vi "Main.vi"() -> ()   [LabVIEW 2020]
doc: "This template is for the Queued Message Handler design pattern.\n\nThe Event Handling Loop generates messages based on user interface actions.\n\nThe Message Handling Loop processes messages generated by the Event Handling Loop, or by other messages. The messages are string values, so new messages can be added easily to the Message Cases case structure in the Message Handling Loop. Each message cluster can also provide an optional value for Message Data, which is a variant that can be converted to whatever message-specific data is required."
uses:
  TrioMotion Controller/Connection Type.ctl
  support/Message Queue/Message Cluster.ctl
  controls/MHL Data.ctl
  controls/MHL UI Data.ctl
  controls/MHL Status.ctl
  controls/MHL References.ctl
  controls/MHL Configuration.ctl
  <extravilib>/ChannelInstances/Messenger-t'Message Queue.lvlib-Message Cluster.ctl'/Write With Abort.vi
  <extravilib>/ChannelInstances/Messenger-t'Message Queue.lvlib-Message Cluster.ctl'/Instantiate.vi
  <extravilib>/ChannelInstances/Messenger-t'Message Queue.lvlib-Message Cluster.ctl'/Endpoint.vi
  <extravilib>/ChannelInstances/Event Messenger-bool/Instantiate.vi
  <extravilib>/ChannelInstances/Event Messenger-bool/))Channel.vi
  <vilib>/Utility/error.llb/Error Cluster From Error Code.vi
  <vilib>/ErrorRing/Error Ring.xnode
  <extravilib>/ChannelInstances/Event Messenger-bool.lvlib
  support/Message Queue/Message Queue.lvlib
  <extravilib>/ChannelInstances/Messenger-t'Message Queue.lvlib-Message Cluster.ctl'.lvlib
  TrioMotion Controller/TrioMotion Controller.lvlib
panel:
  in  "Home Axes":bool
  in  "Enable Axes":bool
  in  "Set Parameters":bool
  in  "Connection Type":T1
  in  "Connect to Controller":bool
  out "Status":string
  in  "Exit":bool
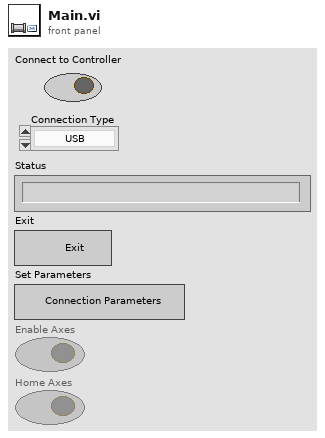
[diagram p1: front panel]
types:
  T1 = typedef "TrioMotion Controller.lvlib/Connection Type.ctl" = enum16{"USB", "Serial", "Ethernet", "PCI", "Path", "No connection"}
  T2 = typedef "MHL Data.ctl" = cluster{"MHL UI Data":T3, "MHL References":T5, "MHL Configuration":T6}
  T3 = typedef "MHL UI Data.ctl" = cluster{"Status":string, "Connection Type":T1, "Connected to Controller":bool, "Axes Enabled":bool, "Jogging Enabled":bool, "X Axis MPOS":dbl, "A Axis MPOS":dbl, "X Axis SPEED":dbl, "A Axis SPEED":dbl, "Plot Laser Data":bool, "MHL Status":T4}
  T4 = typedef "MHL Status.ctl" = enum16{"Disconnected", "Connecting", "Connected", "Axes Enabled", "Machine Running", "Shutdown"}
  T5 = typedef "MHL References.ctl" = cluster{"Connect to Controller Ref":refnum<vi>, "Connection Type Ref":refnum<vi>, "Set Parameters Ref":refnum<vi>, "Enable Axes Ref":refnum<vi>, "Home Axes Ref":refnum<vi>}
  T6 = typedef "MHL Configuration.ctl" = cluster{"Fuel Control Valve Maximum":dbl, "Fuel Control Valve Minimum":dbl}
  T7 = typedef "Message Queue.lvlib/Message Cluster.ctl" = cluster{"Message":string, "Message Data":variant}
  T8 = typedef "Notifiers.ctl" = cluster{"Handshake":refnum<notifier>, "Connection Established":refnum<notifier>, "Controller Exit":refnum<notifier>}
  T9 = typedef "Messenger-t'Message Queue.lvlib-Message Cluster.ctl'.lvlib/))Channel.ctl" = refnum<queue>
  T10 = typedef "Event Messenger-bool.lvlib/))Channel.ctl" = refnum<queue>
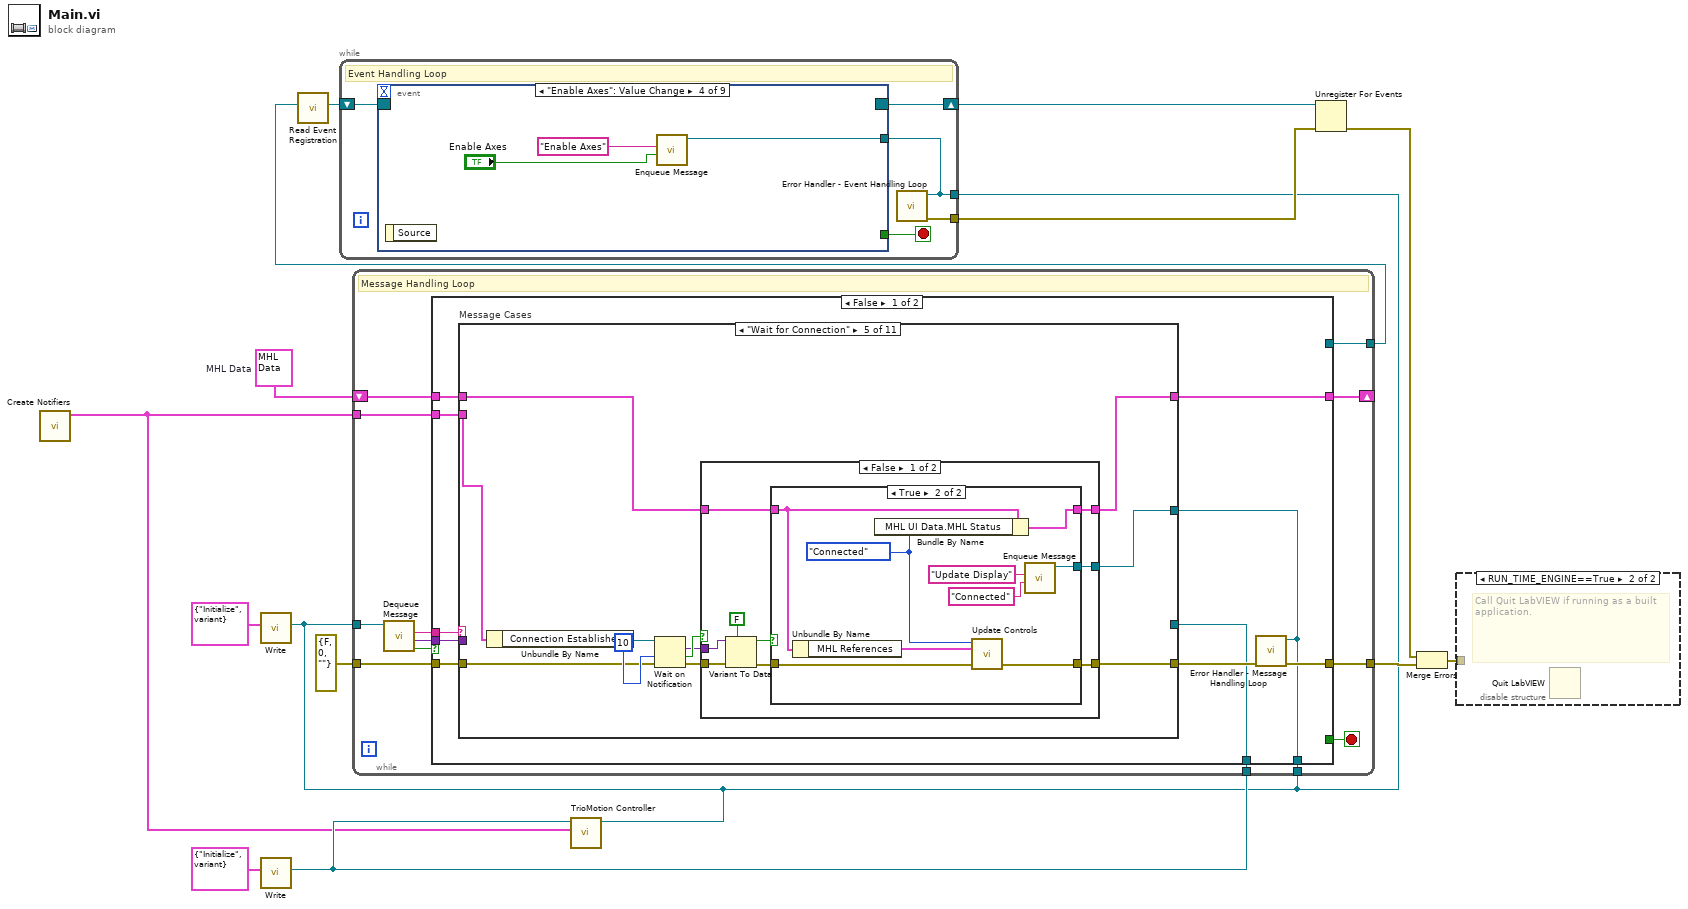
[diagram p0: block diagram]
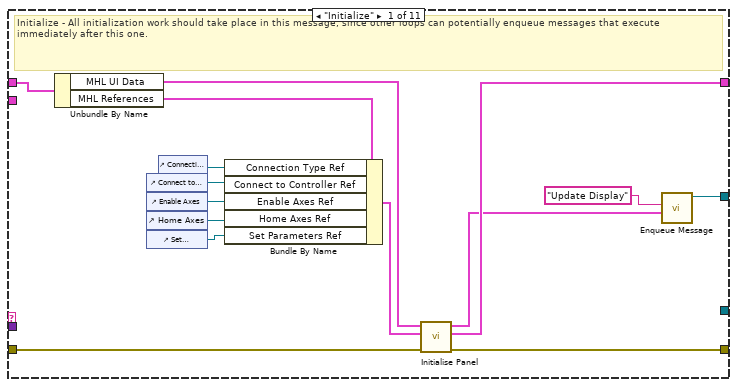
[diagram p2: hidden frame]
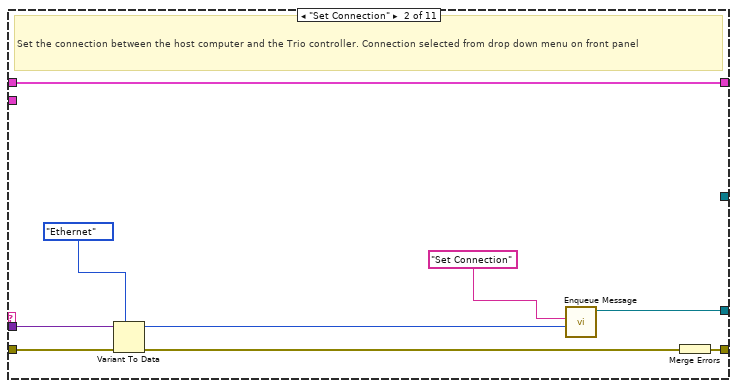
[diagram p3: hidden frame]
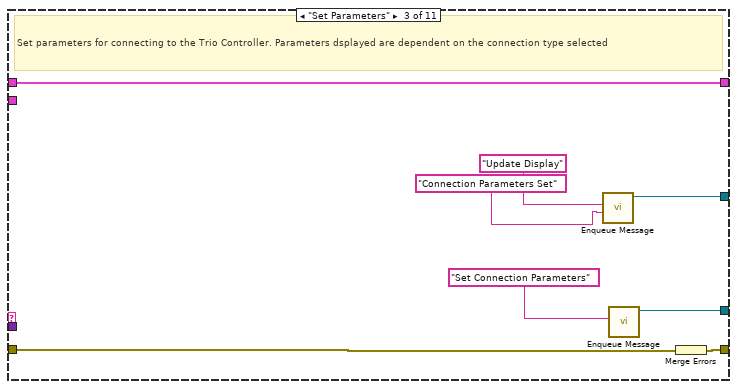
[diagram p4: hidden frame]
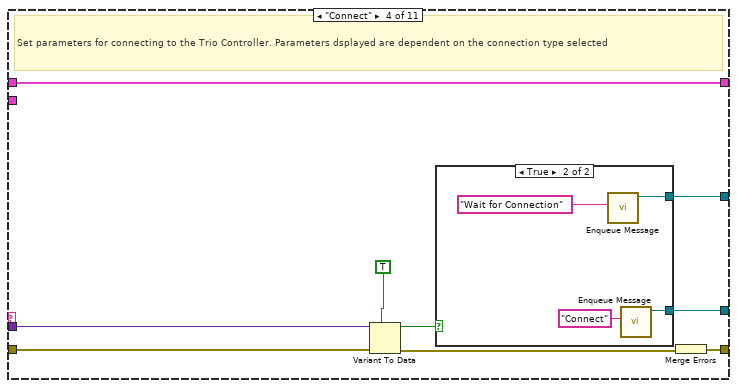
[diagram p5: hidden frame]
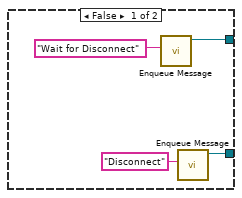
[diagram p6: hidden frame]
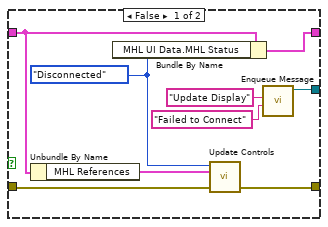
[diagram p7: hidden frame]
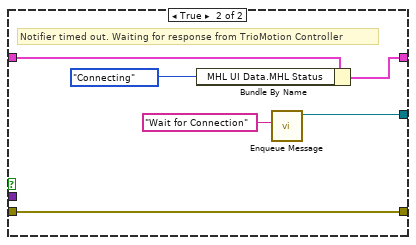
[diagram p8: hidden frame]
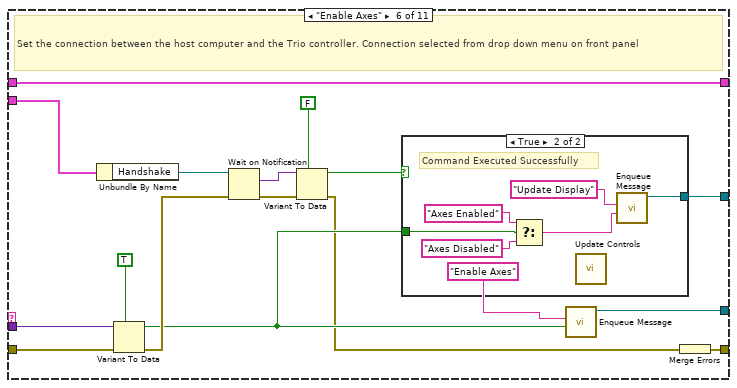
[diagram p9: hidden frame]
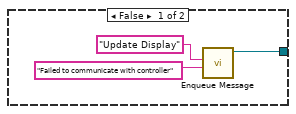
[diagram p10: hidden frame]
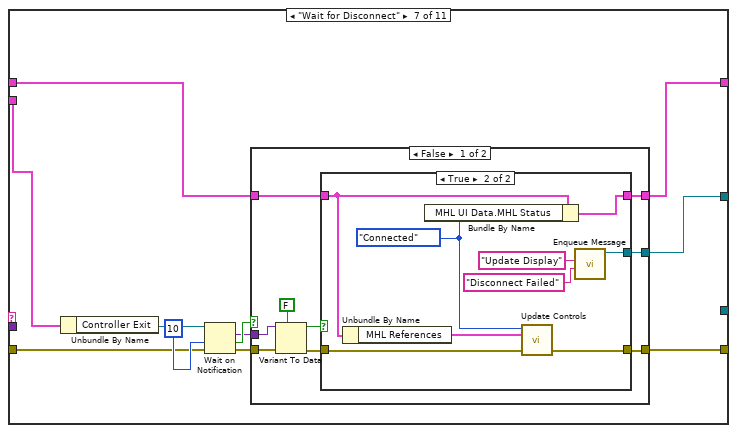
[diagram p11: hidden frame]
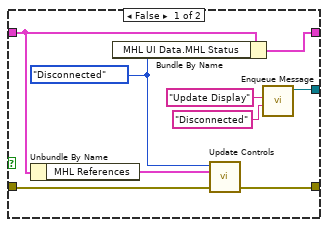
[diagram p12: hidden frame]
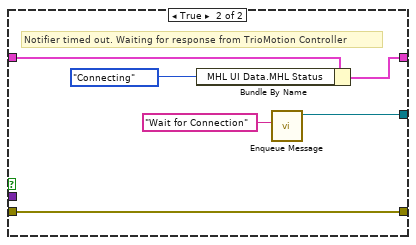
[diagram p13: hidden frame]
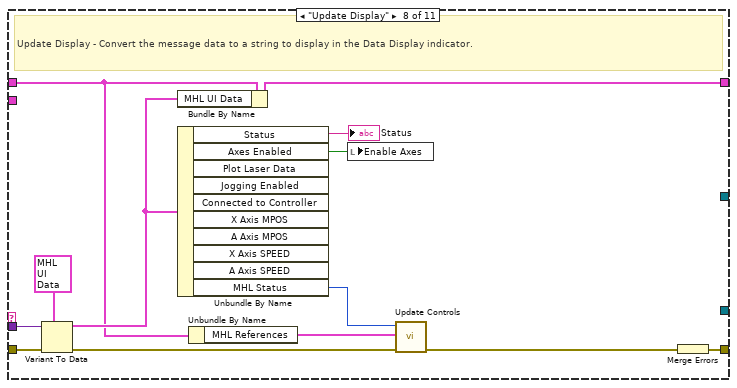
[diagram p14: hidden frame]
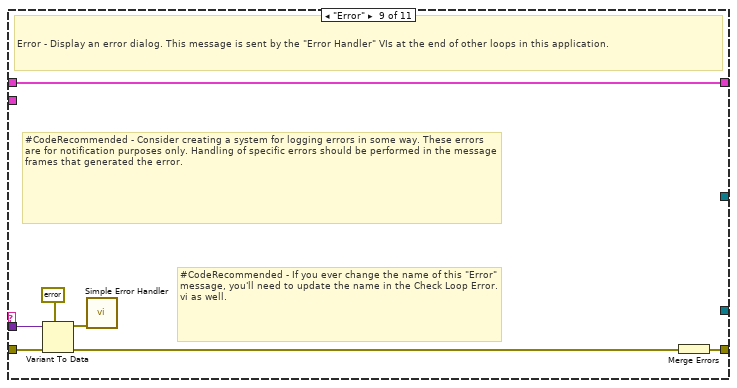
[diagram p15: hidden frame]
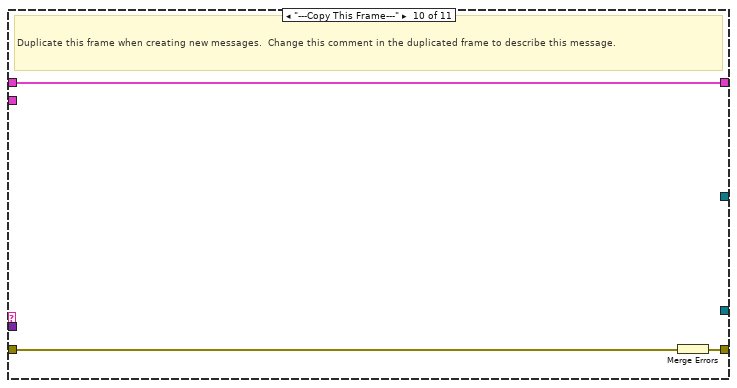
[diagram p16: hidden frame]
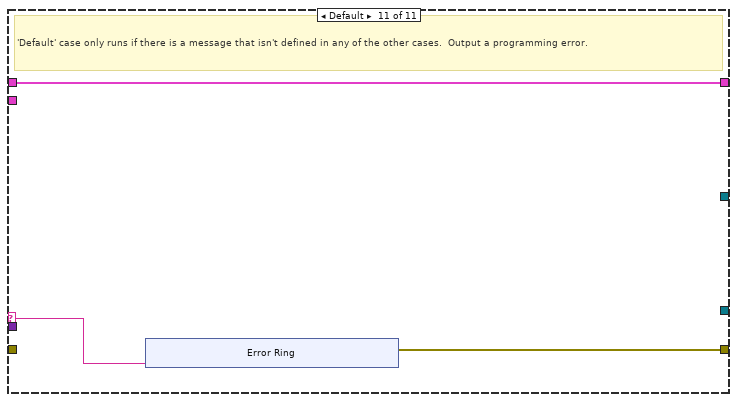
[diagram p17: hidden frame]
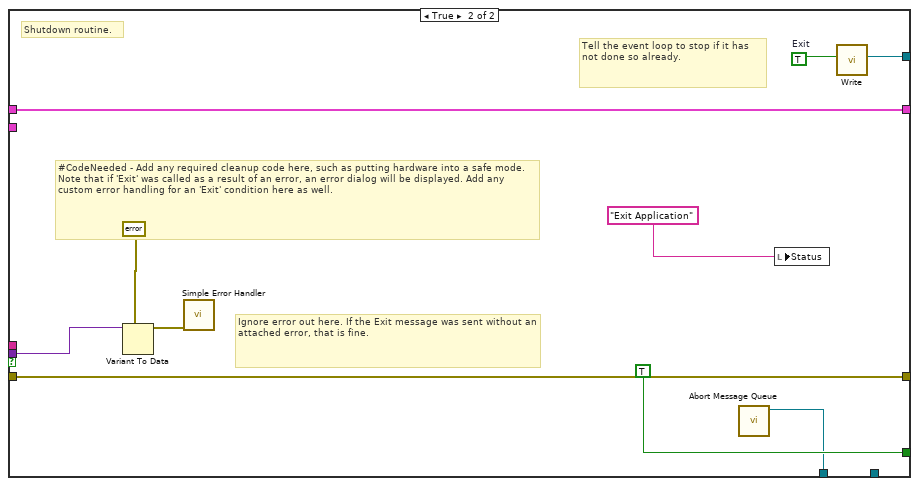
[diagram p18: hidden frame]
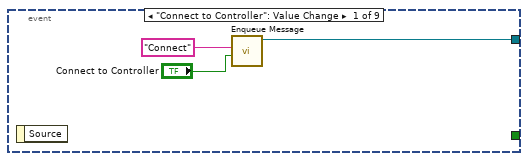
[diagram p20: hidden frame]
diagram:
  w3 = T2 {"MHL UI Data"={"Status"="", "Connection Type"=enum."Ethernet", "Connected to Controller"=FALSE, "Axes Enabled"=FALSE, "Jogging Enabled"=FALSE, "X Axis MPOS"=0.0, "A Axis MPOS"=0.0, "X Axis SPEED"=0.0, "A Axis SPEED"=0.0, "Plot Laser Data"=FALSE, "MHL Status"=enum."Disconnected"}, "MHL References"={"Connect to Controller Ref"=refnum, "Connection Type Ref"=refnum, "Set Parameters Ref"=refnum, "Enable Axes Ref"=refnum, "Home Axes Ref"=refnum}, "MHL Configuration"={"Fuel Control Valve Maximum"=0.0, "Fuel Control Valve Minimum"=0.0}}  # MHL Data
  n1 = call "Create Notifiers.vi"() -> ("Notifiers"=w2:T8)  [unwired: 10 in, 1 out]
  n2 = call <extravilib>:"Write.vi"("element"=T7 {"Message"="Initialize", "Message Data"=variant}) -> ("channel"=w1:T9)  [unwired: 8 in, 2 out]
  n3 = call <extravilib>:"Write.vi"("element"=T7 {"Message"="Initialize", "Message Data"=variant}) -> ("channel"=w4:T9)  [unwired: 8 in, 2 out]
  n4 = while {
    shift-right: [w26] -> _
    shift-left: w3 -> [w27]
    tunnel: [w24] -> w14
    tunnel: [w23] -> w10
    tunnel: w1 -> [w20]
    tunnel: errorcluster {"status"=FALSE, "code"=0, "source"=""} ("error IO") -> [w22]
    tunnel: w1 -> [w21]
    tunnel: w4 -> [w16]
    tunnel: w2 -> [w15]
    stop <- w25 stop-if-true
    # "Message Handling Loop"
    n5 = call "Dequeue Message.vi"("channel"=w20) -> ("channel aborted"=w17:bool, "message data"=w18:variant, "message"=w19:string)  [unwired: 8 in]
    n6 = case shown="False" w17 {
      tunnel: w27 -> [w37 w241]
      tunnel: [w36 w241] -> w26
      tunnel: [_ TRUE] -> w25
      tunnel: [w35 w242] -> w24
      tunnel: [_ w236] -> w23
      tunnel: w19 -> [w33 _]
      tunnel: w18 -> [w32 w238]
      tunnel: w22 -> [w31 w242]
      tunnel: [w30 _] -> w21
      tunnel: [w29 w234] -> w16
      tunnel: w15 -> [w28 _]
      frame False {
        n7 = case "Message Cases" shown="\"Wait for Connection\"" w33 {
          selector: w33 -> [_ _ _ _ _ _ _ _ _ _ w224]
          tunnel: w31 -> [w44 w58 w67 w75 w94 w144 w164 w212 w220 w223 _]
          tunnel: [w43 w60 w68 w77 w87 w146 w157 w213 w214 w221 w225] -> w34
          tunnel: w37 -> [w50 w61 w69 w78 w88 w147 w158 w203 w219 w222 w226]
          tunnel: [w39 w61 w69 w78 w89 w147 w159 w209 w219 w222 w226] -> w36
          tunnel: w32 -> [_ w59 _ w71 _ w145 _ w211 w218 _ _]
          tunnel: [w52 _ w66 w70 w91 w135 w161 _ _ _ _] -> w30
          tunnel: [_ w55 w62 w73 _ w142 _ _ _ _ _] -> w29
          tunnel: w28 -> [_ _ _ _ w97 w141 w167 _ _ _ _]
          frame "Initialize" {
            # "Initialize - All initialization work should take place in this message, since other loops can potentially enqueue messages that execute immediately after this one."
            n8 = Unbundle By Name(w50) -> ("MHL UI Data"=w42:T3, "MHL References"=w49:T5)
            n9 = control-ref of="Connect to Controller"() -> (w48:refnum<vi>)
            n10 = control-ref of="Enable Axes"() -> (w45:refnum<vi>)
            n11 = control-ref of="Home Axes"() -> (w47:refnum<vi>)
            n12 = control-ref of="Set Parameters"() -> (w46:refnum<vi>)
            n13 = control-ref of="Connection Type"() -> (w40:refnum<vi>)
            n14 = Bundle By Name(cluster=w49, "Connection Type Ref"=w40, "Connect to Controller Ref"=w48, "Enable Axes Ref"=w45, "Home Axes Ref"=w47, "Set Parameters Ref"=w46) -> (w41:T5)
            n15 = call "Initialise Panel.vi"("error in"=w44, "MHL References"=w41, "MHL UI Data In"=w42) -> ("error out"=w43:errorcluster, "MHL Data"=w39:T2, "MHL UI Data Out"=w38:T3)  [unwired: 6 in]
            n16 = call "Enqueue Message.vi"("data (empty)"=w38, "message"="Update Display" ("Message")) -> ("channel"=w52:T9)  [unwired: 9 in]
          }
          frame "Set Connection" {
            # "Set the connection between the host computer and the Trio controller. Connection selected from drop down menu on front panel"
            n17 = Variant To Data(error in=w58, type=Connection_Type."Ethernet" ("Connection Method"), Variant=w59) -> (data=w56:T1, error out=w54:errorcluster)
            n18 = call "Enqueue Message.vi"("data (empty)"=w56, "message"="Set Connection" ("Connection Type")) -> ("channel"=w55:T9)  [unwired: 9 in]
            n19 = Merge Errors(w54) -> (w60:errorcluster)
          }
          frame "Set Parameters" {
            # "Set parameters for connecting to the Trio Controller. Parameters dsplayed are dependent on the connection type selected"
            n20 = call "Enqueue Message.vi"("data (empty)"="Connection Parameters Set" ("Initial Message"), "message"="Update Display") -> ("channel"=w66:T9)  [unwired: 9 in]
            n21 = call "Enqueue Message.vi"("message"="Set Connection Parameters") -> ("channel"=w62:T9)  [unwired: 10 in]
            n22 = Merge Errors(w67) -> (w68:errorcluster)
          }
          frame "Connect" {
            # "Set parameters for connecting to the Trio Controller. Parameters dsplayed are dependent on the connection type selected"
            n23 = Variant To Data(error in=w75, type=TRUE, Variant=w71) -> (data=w74:bool, error out=w72:errorcluster)
            n24 = case shown="True" w74 {
              tunnel: [w81 w85] -> w73
              tunnel: [w80 w83] -> w70
              frame False {
                n25 = call "Enqueue Message.vi"("message"="Wait for Disconnect") -> ("channel"=w80:T9)  [unwired: 10 in]
                n26 = call "Enqueue Message.vi"("message"="Disconnect") -> ("channel"=w81:T9)  [unwired: 10 in]
              }
              frame True {
                n27 = call "Enqueue Message.vi"("message"="Wait for Connection") -> ("channel"=w83:T9)  [unwired: 10 in]
                n28 = call "Enqueue Message.vi"("message"="Connect") -> ("channel"=w85:T9)  [unwired: 10 in]
              }
            }
            n29 = Merge Errors(w72) -> (w77:errorcluster)
          }
          frame "Wait for Connection" {
            n30 = Unbundle By Name(w97) -> ("Connection Established"=w96:refnum<notifier>)
            n31 = Wait on Notification(notifier=w96, timeout in ms (-1)=10, error in (no error)=w94) -> (notification=w90:variant, timed out?=w93:bool, error out=w92:errorcluster)  [unwired: 1 in, 1 out]
            n32 = case shown="False" w93 {
              tunnel: w92 -> [w104 w125]
              tunnel: [w102 w129] -> w91
              tunnel: w90 -> [w106 _]
              tunnel: w88 -> [w101 w128]
              tunnel: [w100 w127] -> w89
              tunnel: [w98 w125] -> w87
              frame False {
                n33 = Variant To Data(error in=w104, type=FALSE, Variant=w106) -> (data=w103:bool, error out=w99:errorcluster)
                n34 = case shown="True" w103 {
                  tunnel: [w113 w122] -> w102
                  tunnel: w101 -> [w111 w120]
                  tunnel: [w112 w121] -> w100
                  tunnel: w99 -> [w108 w117]
                  tunnel: [w107 w116] -> w98
                  frame False {
                    w109 = MHL_Status."Disconnected" ("MHL User Interface Data.MHL Status")
                    n35 = Unbundle By Name(w111) -> ("MHL References"=w110:T5)
                    n36 = Bundle By Name(cluster=w111, "MHL UI Data.MHL Status"=w109) -> (w112:T2)
                    n37 = call "Update Controls.vi"("error in"=w108, "MHL References"=w110, "MHL Status"=w109) -> ("error out"=w107:errorcluster)  [unwired: 8 in]
                    n38 = call "Enqueue Message.vi"("data (empty)"="Failed to Connect" ("message"), "message"="Update Display") -> ("channel"=w113:T9)  [unwired: 9 in]
                  }
                  frame True {
                    w118 = MHL_Status."Connected" ("MHL User Interface Data.MHL Status")
                    n39 = Unbundle By Name(w120) -> ("MHL References"=w119:T5)
                    n40 = Bundle By Name(cluster=w120, "MHL UI Data.MHL Status"=w118) -> (w121:T2)
                    n41 = call "Update Controls.vi"("error in"=w117, "MHL References"=w119, "MHL Status"=w118) -> ("error out"=w116:errorcluster)  [unwired: 8 in]
                    n42 = call "Enqueue Message.vi"("data (empty)"="Connected" ("message"), "message"="Update Display") -> ("channel"=w122:T9)  [unwired: 9 in]
                  }
                }
              }
              frame True {
                # "Notifier timed out. Waiting for response from TrioMotion Controller"
                n43 = Bundle By Name(cluster=w128, "MHL UI Data.MHL Status"=MHL_Status."Connecting" ("MHL User Interface Data.MHL Status")) -> (w127:T2)
                n44 = call "Enqueue Message.vi"("message"="Wait for Connection") -> ("channel"=w129:T9)  [unwired: 10 in]
              }
            }
          }
          frame "Enable Axes" {
            # "Set the connection between the host computer and the Trio controller. Connection selected from drop down menu on front panel"
            n45 = Unbundle By Name(w141) -> ("Handshake"=w140:refnum<notifier>)
            n46 = Variant To Data(error in=w144, type=TRUE, Variant=w145) -> (data=w133:bool, error out=w139:errorcluster)
            n47 = Wait on Notification(notifier=w140, error in (no error)=w139) -> (notification=w138:variant, error out=w132:errorcluster)  [unwired: 2 in, 2 out]
            n48 = Variant To Data(error in=w132, type=FALSE, Variant=w138) -> (data=w136:bool, error out=w131:errorcluster)
            n49 = case shown="True" w136 {
              tunnel: [w149 w155] -> w135
              tunnel: w133 -> [_ w152]
              frame False {
                n50 = call "Enqueue Message.vi"("data (empty)"="Failed to communicate with controller" ("Message"), "message"="Update Display" ("Message")) -> ("channel"=w149:T9)  [unwired: 9 in]
              }
              frame True {
                # "Command Executed Successfully"
                n51 = Select(t="Axes Enabled" ("Initial Message"), s=w152, f="Axes Disabled" ("Initial Message")) -> (s? t:f=w151:string)
                n52 = call "Update Controls.vi"() -> ()  [unwired: 11 in, 1 out]
                n53 = call "Enqueue Message.vi"("data (empty)"=w151, "message"="Update Display" ("Message")) -> ("channel"=w155:T9)  [unwired: 9 in]
              }
            }
            n54 = call "Enqueue Message.vi"("data (empty)"=w133, "message"="Enable Axes" ("Connection Type")) -> ("channel"=w142:T9)  [unwired: 9 in]
            n55 = Merge Errors(w131) -> (w146:errorcluster)
          }
          frame "Wait for Disconnect" {
            n56 = Unbundle By Name(w167) -> ("Controller Exit"=w166:refnum<notifier>)
            n57 = Wait on Notification(notifier=w166, timeout in ms (-1)=10, error in (no error)=w164) -> (notification=w160:variant, timed out?=w163:bool, error out=w162:errorcluster)  [unwired: 1 in, 1 out]
            n58 = case shown="False" w163 {
              tunnel: w162 -> [w174 w195]
              tunnel: [w172 w199] -> w161
              tunnel: w160 -> [w176 _]
              tunnel: w158 -> [w171 w198]
              tunnel: [w170 w197] -> w159
              tunnel: [w168 w195] -> w157
              frame False {
                n59 = Variant To Data(error in=w174, type=FALSE, Variant=w176) -> (data=w173:bool, error out=w169:errorcluster)
                n60 = case shown="True" w173 {
                  tunnel: [w183 w192] -> w172
                  tunnel: w171 -> [w181 w190]
                  tunnel: [w182 w191] -> w170
                  tunnel: w169 -> [w178 w187]
                  tunnel: [w177 w186] -> w168
                  frame False {
                    w179 = MHL_Status."Disconnected" ("MHL User Interface Data.MHL Status")
                    n61 = Unbundle By Name(w181) -> ("MHL References"=w180:T5)
                    n62 = Bundle By Name(cluster=w181, "MHL UI Data.MHL Status"=w179) -> (w182:T2)
                    n63 = call "Update Controls.vi"("error in"=w178, "MHL References"=w180, "MHL Status"=w179) -> ("error out"=w177:errorcluster)  [unwired: 8 in]
                    n64 = call "Enqueue Message.vi"("data (empty)"="Disconnected" ("message"), "message"="Update Display") -> ("channel"=w183:T9)  [unwired: 9 in]
                  }
                  frame True {
                    w188 = MHL_Status."Connected" ("MHL User Interface Data.MHL Status")
                    n65 = Unbundle By Name(w190) -> ("MHL References"=w189:T5)
                    n66 = Bundle By Name(cluster=w190, "MHL UI Data.MHL Status"=w188) -> (w191:T2)
                    n67 = call "Update Controls.vi"("error in"=w187, "MHL References"=w189, "MHL Status"=w188) -> ("error out"=w186:errorcluster)  [unwired: 8 in]
                    n68 = call "Enqueue Message.vi"("data (empty)"="Disconnect Failed" ("message"), "message"="Update Display") -> ("channel"=w192:T9)  [unwired: 9 in]
                  }
                }
              }
              frame True {
                # "Notifier timed out. Waiting for response from TrioMotion Controller"
                n69 = Bundle By Name(cluster=w198, "MHL UI Data.MHL Status"=MHL_Status."Connecting" ("MHL User Interface Data.MHL Status")) -> (w197:T2)
                n70 = call "Enqueue Message.vi"("message"="Wait for Connection") -> ("channel"=w199:T9)  [unwired: 10 in]
              }
            }
          }
          frame "Update Display" {
            # "Update Display - Convert the message data to a string to display in the Data Display indicator."
            n71 = Variant To Data(error in=w212, type=T3 {"Status"="", "Connection Type"=enum."Ethernet", "Connected to Controller"=FALSE, "Axes Enabled"=FALSE, "Jogging Enabled"=FALSE, "X Axis MPOS"=0.0, "A Axis MPOS"=0.0, "X Axis SPEED"=0.0, "A Axis SPEED"=0.0, "Plot Laser Data"=FALSE, "MHL Status"=enum."Disconnected"} ("MHL UI Data"), Variant=w211) -> (data=w208:T3, error out=w206:errorcluster)
            n72 = Bundle By Name(cluster=w203, "MHL UI Data"=w208) -> (w209:T2)
            n73 = Unbundle By Name(w208) -> ("Status"=→"Status":string, "Axes Enabled"=w201:bool, "MHL Status"=w204:T4)  [unwired: 7 out]
            n74 = Unbundle By Name(w203) -> ("MHL References"=w202:T5)
            n75 = local write "Enable Axes"(w201) -> ()
            n76 = call "Update Controls.vi"("error in"=w206, "MHL References"=w202, "MHL Status"=w204) -> ("error out"=w205:errorcluster)  [unwired: 8 in]
            n77 = Merge Errors(w205) -> (w213:errorcluster)
          }
          frame "Error" {
            # "#CodeRecommended - If you ever change the name of this \"Error\" message, you'll need to update the name in the Check Loop Error.vi as well."
            # "#CodeRecommended - Consider creating a system for logging errors in some way. These errors are for notification purposes only. Handling of specific errors should be performed in the message frames that generated the error."
            # "Error - Display an error dialog. This message is sent by the \"Error Handler\" VIs at the end of other loops in this application."
            n78 = Variant To Data(error in=w220, type=errorcluster {"status"=FALSE, "code"=0, "source"=""} ("error constant"), Variant=w218) -> (data=w216:errorcluster, error out=w215:errorcluster)
            n79 = call <vilib>:"Simple Error Handler.vi"("error in (no error)"=w216) -> ()  [unwired: 4 in, 5 out]
            n80 = Merge Errors(w215) -> (w214:errorcluster)
          }
          frame "---Copy This Frame---" {
            # "Duplicate this frame when creating new messages.  Change this comment in the duplicated frame to describe this message."
            n81 = Merge Errors(w223) -> (w221:errorcluster)
          }
          frame Default {
            # "'Default' case only runs if there is a message that isn't defined in any of the other cases.  Output a programming error."
            n82 = xnode "Error Ring"("parameter 0"=w224) -> ("error out"=w225:errorcluster)
          }
        }
        n83 = call "Error Handler - Message Handling Loop.vi"("channel"=w30, "error in (no error)"=w34) -> ("dup error in"=w35:errorcluster)  [unwired: 9 in]
      }
      frame True {
        w237 = TRUE  # Exit
        # "Tell the event loop to stop if it has not done so already."
        # "Ignore error out here. If the Exit message was sent without an attached error, that is fine."
        # "#CodeNeeded - Add any required cleanup code here, such as putting hardware into a safe mode. Note that if 'Exit' was called as a result of an error, an error dialog will be displayed. Add any custom error handling for an 'Exit' condition here as well."
        # "Shutdown routine."
        n84 = Variant To Data(type=errorcluster {"status"=FALSE, "code"=0, "source"=""} ("error constant"), Variant=w238) -> (data=w239:errorcluster)  [unwired: 1 in, 1 out]
        n85 = call <vilib>:"Simple Error Handler.vi"("error in (no error)"=w239) -> ()  [unwired: 4 in, 5 out]
        n86 = call "Abort Message Queue.vi"() -> ("channel"=w234:T9)  [unwired: 11 in]
        n87 = local write "Status"("Exit Application" ("Exit Application")) -> ()
        n88 = call <extravilib>:"Write.vi"("element"=w237) -> ("channel"=w236:T10)  [unwired: 9 in, 1 out]
      }
    }
  }
  n89 = call <extravilib>:"Read Event Registration.vi"("channel"=w10) -> ("event registration refnum"=w9:refnum<event-registration>)  [unwired: 10 in]
  n90 = while {
    shift-right: [w247] -> w12
    shift-left: w9 -> [w248]
    tunnel: [w245] -> w11
    tunnel: w1 -> [w244]
    stop <- w246 stop-if-true
    # "Event Handling Loop"
    n91 = event shown="[3] \"Enable Axes\": Value Change" {
      selector: w248 -> [_ _ _ _ _ _ _ _ _]
      dyn-events: [_ _ _ _ _ _ _ _ _] -> w247
      timeout: _ -> [_ _ _ _ _ _ _ _ _]
      tunnel: [_ _ _ _ _ w263 _ w266 TRUE ("Discard?")] -> w246
      tunnel: [w251 w255 w257 w260 w262 w264 _ w267 _] -> w244
      event "Connect to Controller": Value Change {
        n92 = event-data() -> ()  [unwired: 1 in, 1 out]
        n93 = call "Enqueue Message.vi"("data (empty)"="Connect to Controller", "message"="Connect" ("Message")) -> ("channel"=w251:T9)  [unwired: 9 in]
      }
      event Value Change {
        n94 = event-data() -> ()  [unwired: 1 in, 1 out]
        n95 = To Variant(anything="Connection Type") -> (Variant=w252:variant)
        n96 = call "Enqueue Message.vi"("data (empty)"=w252, "message"="Set Connection" ("Message")) -> ("channel"=w255:T9)  [unwired: 9 in]
      }
      event "Set Parameters": Value Change {
        n97 = event-data() -> ()  [unwired: 1 in, 1 out]
        n98 = call "Enqueue Message.vi"("message"="Set Parameters" ("Message")) -> ("channel"=w257:T9)  [unwired: 10 in]
      }
      event "Enable Axes": Value Change {
        n99 = event-data() -> ()  [unwired: 1 in, 1 out]
        n100 = call "Enqueue Message.vi"("data (empty)"="Enable Axes", "message"="Enable Axes" ("Message")) -> ("channel"=w260:T9)  [unwired: 9 in]
      }
      event "Home Axes": Value Change {
        n101 = event-data() -> ()  [unwired: 1 in, 1 out]
        n102 = call "Enqueue Message.vi"("message"="Home Axes" ("Message")) -> ("channel"=w262:T9)  [unwired: 10 in]
      }
      event Panel Close? {
        # "Ask user to confirm quit, which will send the exit message if the user says yes. Regardless of the user's response, discard the event so the Exit message has a chance to run to clean up the application."
        n103 = event-data() -> ()  [unwired: 1 in, 1 out]
        n104 = call "Error Handler - Confirm Quit.vi"() -> ("exit confirmed"=w263:bool, "channel"=w264:T9)  [unwired: 10 in]
        n105 = event-data("Discard?"=TRUE) -> ()  [unwired: 1 in, 1 out]
      }
      event Application Instance Close {
        # "#CodeRecommended - When a project closes, all VIs within that project are aborted and leave memory. However, any code placed in this event frame is guaranteed to run to completion, so add any cleanup code that absolutely must happen here when working in the development environment. Normal shutdown code should go in the \"aborted=true\" frame in the Message Handling Loop."
        n106 = event-data() -> ()  [unwired: 1 in, 1 out]
      }
      event "Exit": Value Change {
        n107 = event-data() -> ()  [unwired: 1 in, 1 out]
        n108 = call "Error Handler - Confirm Quit.vi"() -> ("exit confirmed"=w266:bool, "channel"=w267:T9)  [unwired: 10 in]
      }
      event User Event {
        # "The Message Handling Loop processed an \"Exit\" message, which fired this event to stop the Event Handling Loop."
        n109 = event-data() -> ()  [unwired: 1 in, 1 out]
      }
    }
    n110 = call "Error Handler - Event Handling Loop.vi"("channel"=w244) -> ("dup error in"=w245:errorcluster)  [unwired: 10 in]
  }
  n111 = call "TrioMotion Controller.vi"("channel out"=w1, "Notifiers"=w2, "Channel in"=w4) -> ()  [unwired: 9 in]
  n112 = Unregister For Events(event registration refnum=w12, error in=w11) -> (error out=w13:errorcluster)
  n113 = Merge Errors(w13, w14) -> (w8:errorcluster)
  n114 = disable-structure shown="RUN_TIME_ENGINE==True" {
    disable-tunnel: w8 -> [_ _]
    frame condition #0 (active) {
    }
    frame condition #1 {
      # "Call Quit LabVIEW if running as a built application."
      n115 = Quit LabVIEW() -> ()  [unwired: 1 in]
    }
  }
